vi "Run_message_reader.vi"(1 "Run Message":string) -> (0 "Error Severity":string)   [LabVIEW 2010]
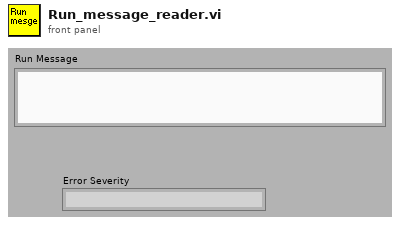
[diagram p1: front panel]
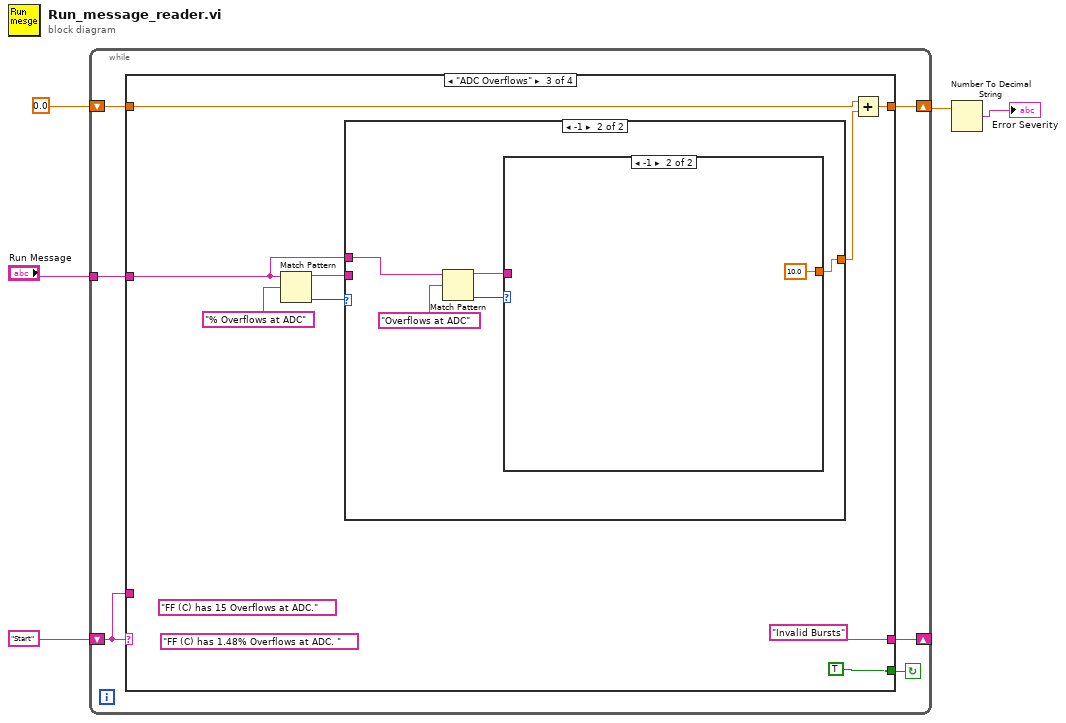
[diagram p0: block diagram]
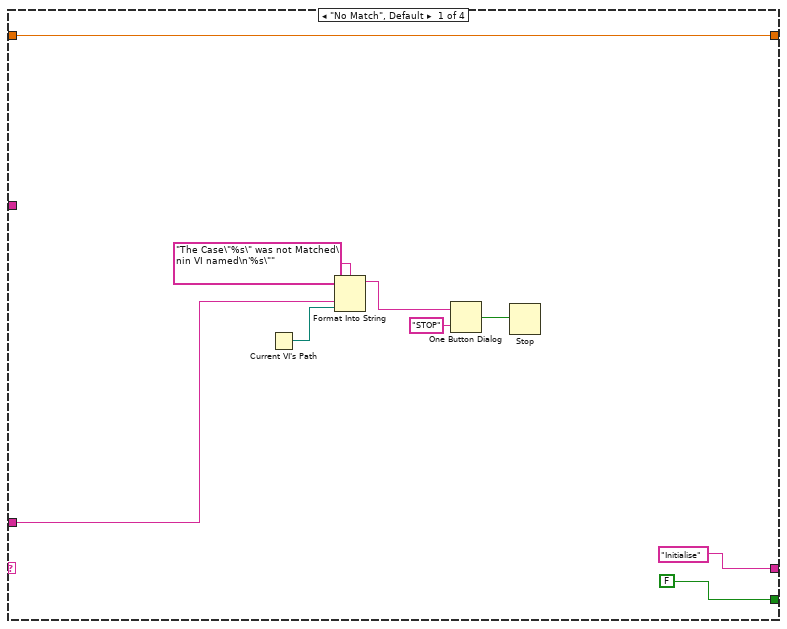
[diagram p2: hidden frame]
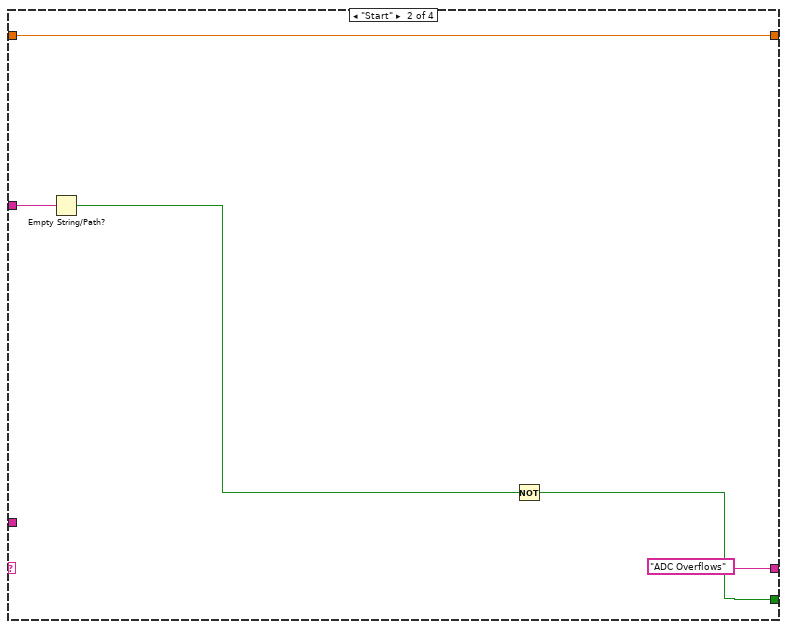
[diagram p3: hidden frame]
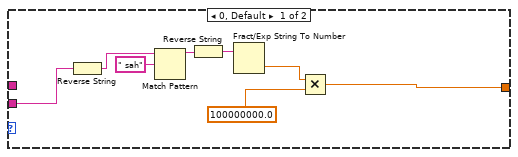
[diagram p4: hidden frame]
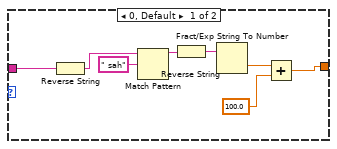
[diagram p5: hidden frame]
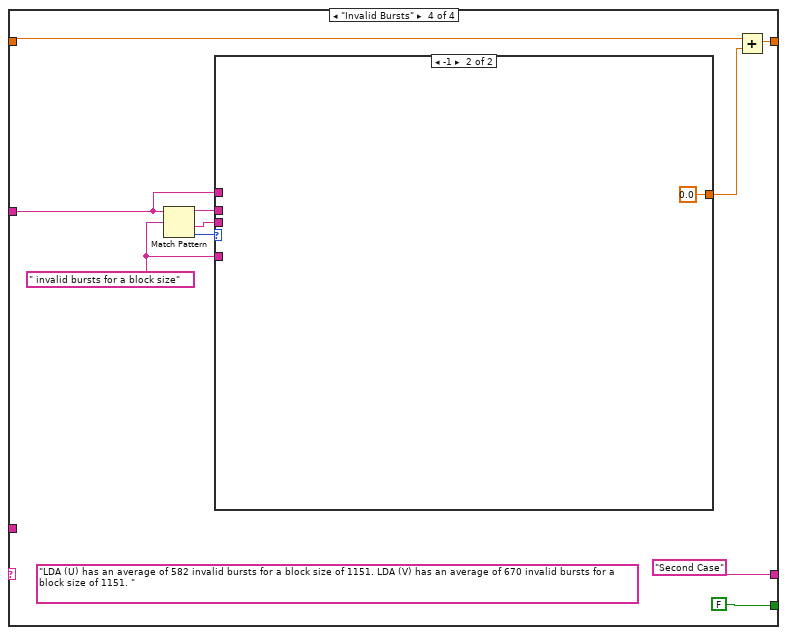
[diagram p6: hidden frame]
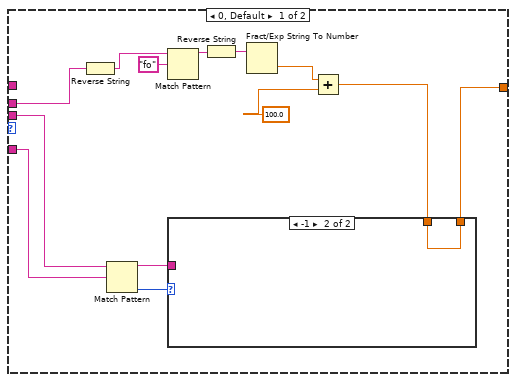
[diagram p7: hidden frame]
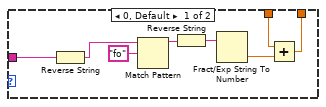
[diagram p8: hidden frame]
diagram:
  n1 = while {
    shift-left: "Start" -> [w9]
    shift-right: [w10] -> _
    tunnel: "Run Message" -> [w8]
    shift-right: [w7] -> w2
    shift-left: 0.0 ("Error Severity") -> [w6]
    stop <- w11 continue-if-true
    n2 = case shown="\"ADC Overflows\"" w9 {
      tunnel: [FALSE w22 TRUE FALSE] -> w11
      tunnel: ["Initialise" "ADC Overflows" "Invalid Bursts" "Second Case"] -> w10
      tunnel: w9 -> [w15 _ _ _]
      tunnel: w8 -> [_ w24 w29 w62]
      tunnel: [w12 w21 w28 w57] -> w7
      tunnel: w6 -> [w12 w21 w26 w58]
      frame "No Match", Default {
        n3 = Current VI's Path() -> (path=w14:path)
        n4 = Format Into String(format string="The Case\"%s\" was not Matched\nin VI named\n'%s\"" ("Format String"), w15, w14) -> (resulting string=w18:string)  [unwired: 2 in, 1 out]
        n5 = One Button Dialog(message=w18, button name ("OK")="STOP") -> (true=w16:bool)
        n6 = Stop(stop? (T)=w16) -> ()
      }
      frame "Start" {
        n7 = Empty String/Path?(string/path=w24) -> (empty?=w23:bool)
        n8 = Not(x=w23) -> (.not. x?=w22:bool)
      }
      frame "ADC Overflows" {
        (unwired) "FF (C) has 15 Overflows at ADC."
        (unwired) "FF (C) has 1.48% Overflows at ADC. "
        n9 = Match Pattern(string=w29, regular expression="% Overflows at ADC") -> (before substring=w30:string, offset past match=w31:i32)  [unwired: 1 in, 2 out]
        n10 = case shown="-1" w31 {
          tunnel: w30 -> [w41 _]
          tunnel: [w35 w43] -> w27
          tunnel: w29 -> [_ w46]
          frame 0, Default {
            n11 = Reverse String(1:w41) -> (0:w40:string)
            n12 = Match Pattern(string=w40, regular expression=" sah") -> (before substring=w39:string)  [unwired: 1 in, 3 out]
            n13 = Reverse String(1:w39) -> (0:w38:string)
            n14 = Fract/Exp String To Number(string=w38) -> (number=w37:dbl)  [unwired: 3 in, 1 out]
            n15 = Multiply(x=w37, y=100000000.0 ("Error Severity")) -> (x*y=w35:dbl)
          }
          frame -1 {
            n16 = Match Pattern(string=w46, regular expression="Overflows at ADC") -> (before substring=w44:string, offset past match=w45:i32)  [unwired: 1 in, 2 out]
            n17 = case shown="-1" w45 {
              tunnel: w44 -> [w51 _]
              tunnel: [w49 10.0] -> w43
              frame 0, Default {
                n18 = Reverse String(1:w51) -> (0:w54:string)
                n19 = Match Pattern(string=w54, regular expression=" sah") -> (before substring=w53:string)  [unwired: 1 in, 3 out]
                n20 = Reverse String(1:w53) -> (0:w52:string)
                n21 = Fract/Exp String To Number(string=w52) -> (number=w50:dbl)  [unwired: 3 in, 1 out]
                n22 = Add(x=w50, y=100.0) -> (x+y=w49:dbl)
              }
              frame -1 {
              }
            }
          }
        }
        n23 = Add(x=w26, y=w27) -> (x+y=w28:dbl)
      }
      frame "Invalid Bursts" {
        (unwired) "LDA (U) has an average of 582 invalid bursts for a block size of 1151. LDA (V) has an average of 670 invalid bursts for a block size of 1151. "
        w60 = " invalid bursts for a block size"
        n24 = Match Pattern(string=w62, regular expression=w60) -> (before substring=w63:string, after substring=w61:string, offset past match=w64:i32)  [unwired: 1 in, 1 out]
        n25 = case shown="-1" w64 {
          tunnel: w63 -> [w78 _]
          tunnel: [w67 0.0] -> w59
          tunnel: w62 -> [_ _]
          tunnel: w61 -> [w70 _]
          tunnel: w60 -> [w69 _]
          frame 0, Default {
            n26 = Reverse String(1:w78) -> (0:w77:string)
            n27 = Match Pattern(string=w70, regular expression=w69) -> (before substring=w71:string, offset past match=w72:i32)  [unwired: 1 in, 2 out]
            n28 = Match Pattern(string=w77, regular expression="fo") -> (before substring=w76:string)  [unwired: 1 in, 3 out]
            n29 = Reverse String(1:w76) -> (0:w75:string)
            n30 = Fract/Exp String To Number(string=w75) -> (number=w74:dbl)  [unwired: 3 in, 1 out]
            n31 = Add(x=w74, y=100.0 ("Error Severity")) -> (x+y=w68:dbl)
            n32 = case shown="-1" w72 {
              tunnel: w71 -> [w83 _]
              tunnel: w68 -> [w81 w88]
              tunnel: [w80 w88] -> w67
              frame 0, Default {
                n33 = Reverse String(1:w83) -> (0:w86:string)
                n34 = Match Pattern(string=w86, regular expression="fo") -> (before substring=w85:string)  [unwired: 1 in, 3 out]
                n35 = Reverse String(1:w85) -> (0:w84:string)
                n36 = Fract/Exp String To Number(string=w84) -> (number=w82:dbl)  [unwired: 3 in, 1 out]
                n37 = Add(x=w81, y=w82) -> (x+y=w80:dbl)
              }
              frame -1 {
              }
            }
          }
          frame -1 {
          }
        }
        n38 = Add(x=w58, y=w59) -> (x+y=w57:dbl)
      }
    }
  }
  n39 = Number To Decimal String(number=w2) -> (decimal integer string=→"Error Severity":string)  [unwired: 1 in]
